vi "Read Content.vi"(8 "Error In":errorcluster, 11 "Contentable In":refnum<class "Contentable.lvclass">) -> (0 "Error Out":errorcluster, 2 "Content":string, 3 "Contentable Out":refnum<class "Contentable.lvclass">)   [LabVIEW 2018, in "Toolkit.lvlib" / "Tokens.lvlib" / "Contentable.lvclass"]
doc: "Gets the content of the token. The content is all text that does not include any tags, delimiters, or keys."
uses:
  Contentable.lvclass
  Contentable.lvclass/Contentable.ctl
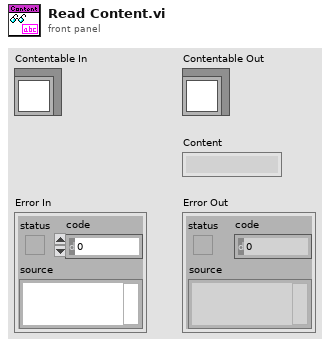
[diagram p1: front panel]
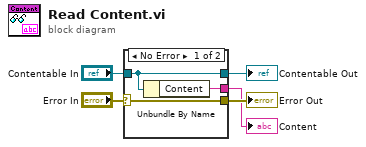
[diagram p0: block diagram]
diagram:
  n1 = case shown="No Error" "Error In" {
    selector: "Error In" -> [w8 w10]
    tunnel: [w8 w10] -> w4
    tunnel: [w7 w9] -> w2
    tunnel: "Contentable In" -> [w7 w9]
    tunnel: [w6 _] -> w1
    frame No Error {
      n2 = Unbundle By Name(w7) -> ("Content"=w6:string)
    }
    frame Error {
    }
  }
  "Error Out" <- w4
  "Contentable Out" <- w2
  "Content" <- w1
